vi "MT Apply Selective Fading Profile.vi"(0 "input complex waveform":T1={"t0"=0.0, "dt"=1.0, "Y"=[]} {"Y" format="%.3f"; "dt" format="%^.2e"; "t0" format="%.4f"}, 5 "fading profile":cdb[][](array[numeric]) format="%.2f", 7 "power delay profile":dbl[][](array[numeric])=[[0.0, 0.0]], 11 "error in (no error)":errorcluster, 13 "reset? (T)":bool=TRUE) -> (4 "output complex waveform":T1 {"Y" format="%.3f"; "dt" format="%^.2e"; "t0" format="%.4f"}, 15 "error out":errorcluster)   [LabVIEW 2020, in "niDMT.lvlib"]
doc: "Applies a multipath fading profile to the <B>input complex waveform</B>."
uses:
  <vilib>/addons/Modulation/niDMT.lvlib
  <vilib>/addons/Modulation/Analog/controls/Complex Data Waveform.ctl
  <vilib>/Analysis/baseanly.llb/Mean (DBL).vi
  <vilib>/addons/Modulation/niAMT.lvlib
  <vilib>/Analysis/NI_AALBase.lvlib
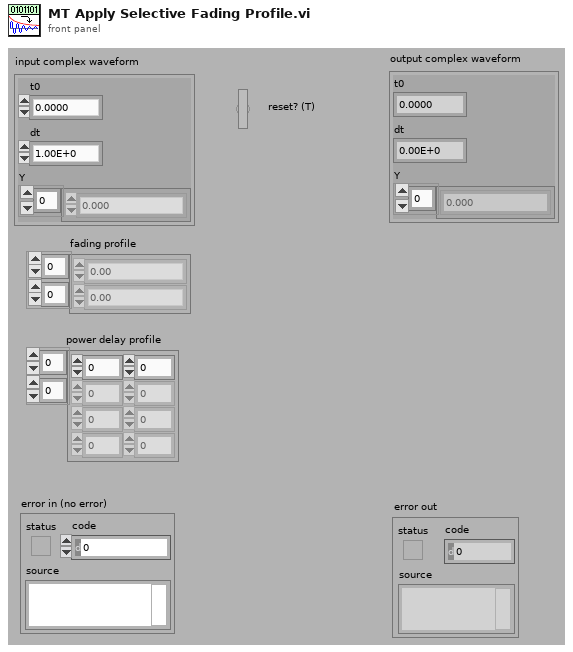
[diagram p1: front panel]
types:
  T1 = typedef "niAMT.lvlib/Complex Data Waveform.ctl" = cluster{"t0":dbl, "dt":dbl, "Y":cdb[]}
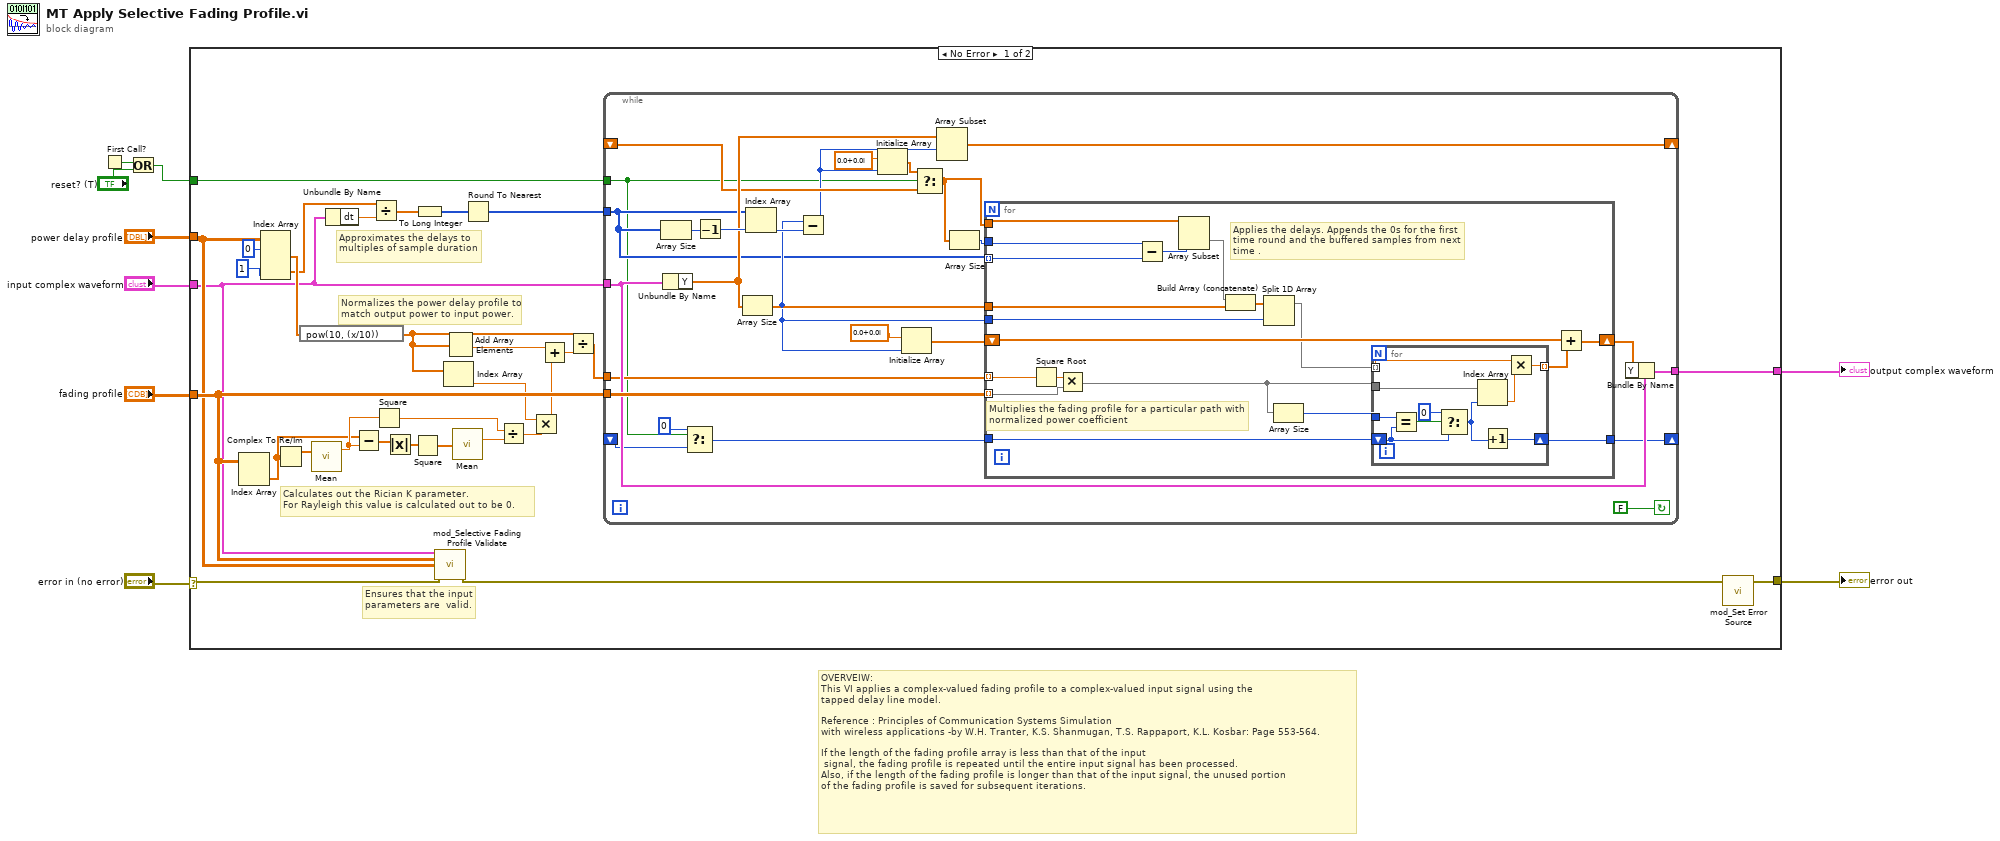
[diagram p0: block diagram]
diagram:
  # "OVERVEIW:\nThis VI applies a complex-valued fading profile to a complex-valued input signal using the \ntapped delay line model. \n\nReference : Principles of Communication Systems Simulation\nwith wireless applications -by W.H. Tranter, K.S. Shanmugan, T.S. Rappaport, K.L. Kosbar: Page 553-564. \n\nIf the length of the fading profile array is less than that of the input\n signal, the fading profile is repeated until the entire input signal has been processed.\nAlso, if the length of the fading profile is longer than that of the input signal, the unused portion\nof the fading profile is saved for subsequent iterations."
  n1 = First Call?() -> (First Call?: T/F=w5:bool)
  n2 = Or(x=w5, y="reset? (T)") -> (x .or. y?=w4:bool)
  n3 = case shown="No Error" "error in (no error)" {
    selector: "error in (no error)" -> [w16 w96]
    tunnel: "input complex waveform" -> [w17 _]
    tunnel: "fading profile" -> [w31 _]
    tunnel: w4 -> [w12 _]
    tunnel: [w40 _] -> w6
    tunnel: [w39 w96] -> w7
    tunnel: "power delay profile" -> [w18 _]
    frame No Error {
      # "Calculates out the Rician K parameter.\nFor Rayleigh this value is calculated out to be 0."
      # "Normalizes the power delay profile to match output power to input power."
      # "Approximates the delays to multiples of sample duration"
      # "Ensures that the input parameters are  valid."
      n4 = Index Array(array=w31) -> (element=w13:cdb[])  [unwired: 2 in]
      n5 = Index Array(array=w18, index (col) #1=0 ("index (row)"), index (col) #2=1 ("index (row)")) -> (element #1=w33:dbl[], element #2=w15:dbl[])  [unwired: 2 in]
      n6 = Complex To Re/Im(x + iy=w13) -> (x=w14:dbl[])  [unwired: 1 out]
      n7 = expression code="pow(10, (x/10))"(w33) -> (w23:dbl[])
      n8 = call-poly <vilib>:"Mean.vi"("X"=w14) -> ("mean"=w29:dbl)  [unwired: 1 out]
      n9 = Unbundle By Name(w17) -> ("dt"=w35:dbl)
      n10 = Subtract(x=w13, y=w29) -> (x-y=w28:cdb[])
      n11 = Divide(x=w15, y=w35) -> (x/y=w38:dbl[])
      n12 = Square(x=w29) -> (x^2=w24:dbl)
      n13 = Absolute Value(x=w28) -> (abs(x)=w27:dbl[])
      n14 = Square(x=w27) -> (x^2=w26:dbl[])
      n15 = To Long Integer(number=w38) -> (32bit integer=w10:i32[])
      n16 = call <vilib>:"mod_Selective Fading Profile Validate.vi"("input complex waveform"=w17, "fading profile"=w31, "power delay profile"=w18, "error in (no error)"=w16) -> ("error out"=w36:errorcluster)  [unwired: 11 out]
      n17 = Index Array(array=w23) -> (element=w22:dbl)  [unwired: 1 in]
      n18 = Add Array Elements(numeric array=w23) -> (sum=w11:dbl)
      n19 = call-poly <vilib>:"Mean.vi"("X"=w26) -> ("mean"=w25:dbl)  [unwired: 1 out]
      n20 = Round To Nearest(number=w10) -> (nearest integer value=w37:i32[])
      n21 = Divide(x=w24, y=w25) -> (x/y=w21:dbl)
      n22 = Multiply(x=w22, y=w21) -> (x*y=w20:dbl)
      n23 = Add(x=w11, y=w20) -> (x+y=w30:dbl)
      n24 = Divide(x=w23, y=w30) -> (x/y=w32:dbl[])
      n25 = while {
        tunnel: [w66] -> w40
        tunnel: w31 -> [w65]
        tunnel: w17 -> [w64]
        tunnel: w32 -> [w63]
        tunnel: w37 -> [w50]
        tunnel: w12 -> [w46]
        shift-right: [w55] -> _
        shift-left: _ -> [w48]
        shift-right: [w52] -> _
        shift-left: _ -> [w45]
        stop <- FALSE continue-if-true
        n26 = Array Size(array=w50) -> (size(s)=w58:i32)
        n27 = Unbundle By Name(w64) -> ("Y"=w56:cdb[])
        n28 = Select(t=0, s=w46, f=w45) -> (s? t:f=w43:i32)
        n29 = Decrement(x=w58) -> (x-1=w59:i32)
        n30 = Array Size(array=w56) -> (size(s)=w53:i32)
        n31 = Index Array(array=w50, index=w59) -> (element=w57:i32)
        n32 = Subtract(x=w53, y=w57) -> (x-y=w47:i32)
        n33 = Initialize Array(cdb 0.0+0.0i ("element"), w47) -> (w49:cdb[])
        n34 = Initialize Array(cdb 0.0+0.0i ("element"), w53) -> (w61:cdb[])
        n35 = Select(t=w49, s=w46, f=w48) -> (s? t:f=w42:cdb[])
        n36 = Array Subset(array=w56, index=w47) -> (w55:cdb[])  [unwired: 1 in]
        n37 = Array Size(array=w42) -> (size(s)=w41:i32)
        n38 = for {
          tunnel: w56 -> [w82]
          tunnel: w65 -> [w78] mode=indexing
          shift-right: [w79] -> w62
          shift-left: w61 -> [w77]
          tunnel: w63 -> [w85] mode=indexing
          tunnel: w50 -> [w68] mode=indexing
          tunnel: w42 -> [w76]
          tunnel: w53 -> [w75]
          tunnel: [w73] -> w52
          tunnel: w43 -> [w72]
          tunnel: w41 -> [w67]
          # "Multiplies the fading profile for a particular path with normalized power coefficient"
          # "Applies the delays. Appends the 0s for the first time round and the buffered samples from next time ."
          n39 = Square Root(x=w85) -> (sqrt(x)=w84:dbl)
          n40 = Multiply(x=w84, y=w78) -> (x*y=w71:cdb[])
          n41 = Subtract(x=w67, y=w68) -> (x-y=w69:i32)
          n42 = Array Subset(array=w76, index=w69) -> (w83:cdb[])  [unwired: 1 in]
          n43 = Build Array (concatenate)(w83, w82) -> (w81:cdb[])
          n44 = Split 1D Array(array=w81, index=w75) -> (first subarray=w74:cdb[])  [unwired: 1 out]
          n45 = Array Size(array=w71) -> (size(s)=w70:i32)
          n46 = for {
            tunnel: [w95] -> w80 mode=indexing
            tunnel: w71 -> [w93]
            tunnel: w74 -> [w86] mode=indexing
            shift-right: [w88] -> w73
            shift-left: w72 -> [w90]
            tunnel: w70 -> [w87]
            n47 = Equal?(x=w87, y=w90) -> (x = y?=w92:bool)
            n48 = Select(t=0, s=w92, f=w90) -> (s? t:f=w89:i32)
            n49 = Index Array(array=w93, index=w89) -> (element=w94:cdb)
            n50 = Increment(x=w89) -> (x+1=w88:i32)
            n51 = Multiply(x=w86, y=w94) -> (x*y=w95:cdb)
          }
          n52 = Add(x=w77, y=w80) -> (x+y=w79:cdb[])
        }
        n53 = Bundle By Name(cluster=w64, "Y"=w62) -> (w66:T1)
      }
      n54 = call <vilib>:"mod_Set Error Source.vi"("final error in (no error)"=w36) -> ("error out"=w39:errorcluster)  [unwired: 2 in, 2 out]
    }
    frame Error {
    }
  }
  "error out" <- w7
  "output complex waveform" <- w6
